vi "题目6.6.vi"() -> ()   [LabVIEW 2017]
panel:
  out "字符串":string
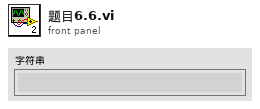
[diagram p1: front panel]
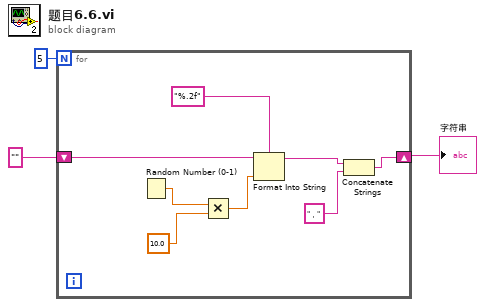
[diagram p0: block diagram]
diagram:
  n1 = for {
    N: 5 -> [_]
    shift-right: [w7] -> w1
    shift-left: "" -> [w9]
    n2 = Random Number (0-1)() -> (number: 0 to 1=w6:dbl)
    n3 = Multiply(x=w6, y=10.0) -> (x*y=w11:dbl)
    n4 = Format Into String(format string="%.2f" ("格式字符串"), initial string=w9, w11) -> (resulting string=w8:string)  [unwired: 1 in, 1 out]
    n5 = Concatenate Strings(w8, "，" ("字符串")) -> (w7:string)
  }
  "字符串" <- w1
